vi "FPGANic-Tester.vi"() -> ()   [LabVIEW 2017]
uses:
  Source.Machine.Settings.ctl
  FPGANic.Events.ctl
  <vilib>/FPGAPlugInAG/PXIe-6592R/niLvFpga_Open_PXIe-6592R.vi
  <vilib>/rvi/interface/common/dynamic/niFpgaDynamicAddResources.vi
  <vilib>/FPGAPlugInAG/Dynamic/niLvFpga_Download_Dynamic.vi
  <vilib>/Utility/error.llb/Error Cluster From Error Code.vi
  <vilib>/rvi/errors/niLvFpgaAdjustHostInterfaceError.vi
  <vilib>/FPGAPlugInAG/Dynamic/niLvFpga_Run_Dynamic.vi
  FPGANic.Globals.vi
  <vilib>/FPGAPlugInAG/Dynamic/niLvFpga_Close_Dynamic.vi
  <vilib>/rvi/interface/nirviOpenFPGA/nirviOpenFPGA.xnode
  ProjectExportForVivado/fpga_nic/fpga_nic.lvbitx
  <vilib>/rvi/interface/nirviMethod/nirviMethod.xnode
  <vilib>/rvi/interface/nirviReadWriteControl/nirviReadWriteControl.xnode
  <vilib>/rvi/interface/nirviCloseFPGA/nirviCloseFPGA.xnode
  <vilib>/FPGAPlugInAG/Dynamic/niLvFpga_ReadFifo_Dynamic.vi
  <vilib>/rvi/errors/niLvFpgaMergeErrorWithErrorCode.vi
  <vilib>/FPGAPlugInAG/Dynamic/niLvFpga_WriteFifo_Dynamic.vi
  NiFpgaLv.dll
  <vilib>/rvi/interface/Simulation/niFpgaSimulationCallBeginRW.vi
panel:
  in  "Polling?":bool
  in  "Clear":bool
  in  "Read UART":bool
  in  "Tab Control":T1(tab)=enum."Probes/GPIO"
  in  "Ethernet II Params":T2={"Destination MAC"=[0, 2, 201, 85, 8, 68], "Source MAC"=[0, 1, 2, 3, 4, 5], "EtherType"=2048} {"Destination MAC" format="%.0x"; "Source MAC" format="%.02x"; "EtherType" format="%.0x"}
  in  "IPv4 Params":T3={"Destination IP"=[10, 0, 1, 100], "Source IP"=[10, 0, 1, 101], "Protocol"=17}
  in  "UDP Params":T4={"Source Port"=35312, "Destination Port"=35312, "Payload"="ABCD"}
  in  "MAC & IP":T5={"MAC Address"=[0, 1, 2, 3, 4, 5], "IP Address"=[10, 0, 1, 101]} {"MAC Address" format="%.0x"}
  out "Write Probe 2":u64[](array[numeric]) format="%.0x"
  out "Write Probe 1":u64[](array[numeric]) format="%.0x"
  out "Read Probe":u64[](array[numeric])=[11817445486661492224, 11817446517453291522, 11817445490022484036, 11817446517571077376, 11817445486650471966, 11817446518510649105, 11817445488139373056, 11817446517460230144, 11817445486661145833, 11817446517787656260, 11817445487417098240, 11817446519651434496, 11817445486644756480, 11817446517436909932, 11817445488513474924, 11817446519188976500, 11817445486735683427, 11817446519071309824, 11817445486669857024, 11817446517436872704, 11817445486712455169, 11817446519127149568, 11817445487441608960, 11817446517436872704, 11817445486741163008, 11817445692824123692, 11817726961621401602, 11817445490939658239, 11817446521731743746, 11817445490022484036, 11817446517571452929, 11817445486778910212, 11817446517436907522, 11817445490022484036, 11817446517604614500, 11817445486644690944, 11817446517436880915, 11817445488902144000, 11817446517436841984, 11817445486644690944, 11817446517436841984, 11817445486644690944, 11817445488835018955, 11817726961621401602, 11817445490939658239, 11817446521731743746, 11817445490022484036, 11817446517571452929, 11817445486778910212, 11817446517436907522, 11817445490022484036, 11817446517604614500, 11817445486644690944, 11817446517436895620, 11817445489682350080, 11817446517436841984, 11817445486644690944, 11817446517436841984, 11817445486644690944, 11817445488759354791, 11817726961621401602, 11817445490939658239, 11817446521731743746, 11817445490022484036, 11817446517571452929, 11817445486778910212, 11817446517436907522, 11817445490022484036, 11817446517604614500, 11817445486644690944, 11817446517436880915, 11817445488902144000, 11817446517436841984, 11817445486644690944, 11817446517436841984, 11817445486644690944, 11817445488835018955, 11817726961621401602, 11817445490939658239, 11817446521731743746, 11817445490022484036, 11817446517571452929, 11817445486778910212, 11817446517436907522, 11817445490022484036, 11817446517604614500, 11817445486644690944, 11817446517436878035, 11817445489493540864, 11817446517436841984, 11817445486644690944, 11817446517436841984, 11817445486644690944, 11817445489115705299, 11817726961621401602, 11817445490939658239, 11817446521731743746, 11817445490022484036, 11817446517571452929, 11817445486778910212, 11817446517436907522, 11817445490022484036, 11817446517604614500, 11817445486644690944, 11817446517436880915, 11817445488902144000, 11817446517436841984, 11817445486644690944, 11817446517436841984, 11817445486644690944, 11817445488835018955, 11817726961621401602, 11817445490939658239, 11817446521731743746, 11817445490022484036, 11817446517571452929, 11817445486778910212, 11817446517436907522, 11817445490022484036, 11817446517604614500, 11817445486644690944, 11817446517436878035, 11817445489493540864, 11817446517436841984, 11817445486644690944, 11817446517436841984, 11817445486644690944, 11817445489115705299, 11817726961621401602, 11817445490939658239, 11817446521731743746, 11817445490022484036, 11817446517571452929, 11817445486778910212, 11817446517436907522, 11817445490022484036, 11817446517604614500, 11817445486644690944, 11817446517436878035, 11817445489493540864, 11817446517436841984, 11817445486644690944, 11817446517436841984, 11817445486644690944, 11817445489115705299, 11817726961621401602, 11817445490939658239, 11817446521731743746, 11817445490022484036, 11817446517571452929, 11817445486778910212, 11817446517436907522, 11817445490022484036, 11817446517604614500, 11817445486644690944, 11817446517436880915, 11817445488902144000, 11817446517436841984, 11817445486644690944, 11817446517436841984, 11817445486644690944, 11817445488835018955, 11817726961621401602, 11817445486661492224, 11817446517453291522, 11817445490022484036, 11817446517571077376, 11817445486650474301, 11817446518510649105, 11817445487986346496, 11817446517460230144, 11817445486661145833, 11817446517787656260, 11817445487417098240, 11817446519651434496, 11817445486644756480, 11817446517436909932, 11817445488513474924, 11817446519188976500, 11817445486735683427, 11817446519071309824, 11817445486669857024, 11817446517436872704, 11817445486712455169, 11817446519127149568, 11817445487441608960, 11817446517436872704, 11817445486741163008, 11817445692824141017, 11817726961621401602, 11817445490939658239, 11817446521731743746, 11817445490022484036, 11817446517571452929, 11817445486778910212, 11817446517436907522, 11817445490022484036, 11817446517604614500, 11817445486644690944, 11817446517436878035, 11817445489493540864, 11817446517436841984, 11817445486644690944, 11817446517436841984, 11817445486644690944, 11817445489115705299, 11817726961621401602, 11817445490939658239, 11817446521731743746, 11817445490022484036, 11817446517571452929, 11817445486778910212, 11817446517436907522, 11817445490022484036, 11817446517604614500, 11817445486644690944, 11817446517436859339, 11817445486682636288, 11817446517436841984, 11817445486644690944, 11817446517436841984, 11817445486644690944, 11817445488555902218, 11817726961621401602, 11817445490939658239, 11817446521731743746, 11817445490022484036, 11817446517571452929, 11817445486778910212, 11817446517436907522, 11817445490022484036, 11817446517604614500, 11817445486644690944, 11817446517436859339, 11817445486682636288, 11817446517436841984, 11817445486644690944, 11817446517436841984, 11817445486644690944, 11817445488555902218, 11817726961621401602, 11817445490939658239, 11817446521731743746, 11817445490022484036, 11817446517571452929, 11817445486778910212, 11817446517436907522, 11817445490022484036, 11817446517604614500, 11817445486644690944, 11817446517436878035, 11817445489493540864, 11817446517436841984, 11817445486644690944, 11817446517436841984, 11817445486644690944, 11817445489115705299, 11817726961621401602, 11817445490939658239, 11817446521731743746, 11817445490022484036, 11817446517571452929, 11817445486778910212, 11817446517436907522, 11817445490022484036, 11817446517604614500, 11817445486644690944, 11817446517436878035, 11817445489493540864, 11817446517436841984, 11817445486644690944, 11817446517436841984, 11817445486644690944, 11817445489115705299, 11817726961621401602, 11817445490939658239, 11817446521731743746, 11817445490022484036, 11817446517571452929, 11817445486778910212, 11817446517436907522, 11817445490022484036, 11817446517604614500, 11817445486644690944, 11817446517436859339, 11817445486682636288, 11817446517436841984, 11817445486644690944, 11817446517436841984, 11817445486644690944, 11817445488555902218, 11817726961621401602, 11817445490939658239, 11817446521731743746, 11817445490022484036, 11817446517571452929, 11817445486778910212, 11817446517436907522, 11817445490022484036, 11817446517604614500, 11817445486644690944, 11817446517436859339, 11817445486682636288, 11817446517436841984, 11817445486644690944, 11817446517436841984, 11817445486644690944, 11817445488555902218, 11817726961621401602, 11817445490939658239, 11817446521731743746, 11817445490022484036, 11817446517571452929, 11817445486778910212, 11817446517436907522, 11817445490022484036, 11817446517604614500, 11817445486644690944, 11817446517436844075, 11817445488075145216, 11817446517436841984, 11817445486644690944, 11817446517436841984, 11817445486644690944, 11817445490337402917, 11817726961621401602, 11817445490939658239, 11817446521731743746, 11817445490022484036, 11817446517571452929, 11817445486778910212, 11817446517436907522, 11817445490022484036, 11817446517604614500, 11817445486644690944, 11817446517436859339, 11817445486682636288, 11817446517436841984, 11817445486644690944, 11817446517436841984, 11817445486644690944, 11817445488555902218, 11817726961621401602, 11817445490939658239, 11817446521731743746, 11817445490022484036, 11817446517571452929, 11817445486778910212, 11817446517436907522, 11817445490022484036, 11817446517604614500, 11817445486644690944, 11817446517436844075, 11817445488075145216, 11817446517436841984, 11817445486644690944, 11817446517436841984, 11817445486644690944, 11817445490337402917, 11817726961621401602, 11817445490939658239, 11817446521731743746, 11817445490022484036, 11817446517571452929, 11817445486778910212, 11817446517436907522, 11817445490022484036, 11817446517604614500, 11817445486644690944, 11817446517436859339, 11817445486682636288, 11817446517436841984, 11817445486644690944, 11817446517436841984, 11817445486644690944, 11817445488555902218, 11817726961621401602, 11817445490939658239, 11817446521731743746, 11817445490022484036, 11817446517571452929, 11817445486778910212, 11817446517436907522, 11817445490022484036, 11817446517604614500, 11817445486644690944, 11817446517436844075, 11817445488075145216, 11817446517436841984, 11817445486644690944, 11817446517436841984, 11817445486644690944, 11817445490337402917, 11817726961621401602, 11817445490939658239, 11817446521731743746, 11817445490022484036, 11817446517571452929, 11817445486778910212, 11817446517436907522, 11817445490022484036, 11817446517604614500, 11817445486644690944, 11817446517436844075, 11817445488075145216, 11817446517436841984, 11817445486644690944, 11817446517436841984, 11817445486644690944, 11817445490337402917, 11817726961621401602, 11817445490939658239, 11817446521731743746, 11817445490022484036, 11817446517571452929, 11817445486778910212, 11817446517436907522, 11817445490022484036, 11817446517604614500, 11817445486644690944, 11817446517436880915, 11817445488905814016, 11817446517436841984, 11817445486644690944, 11817446517436841984, 11817445486644690944, 11817445487441373583, 11817726961621401602, 11817445490939658239, 11817446521731743746, 11817445490022484036, 11817446517571452929, 11817445486778910212, 11817446517436907522, 11817445490022484036, 11817446517604614500, 11817445486644690944, 11817446517436844075, 11817445488075145216, 11817446517436841984, 11817445486644690944, 11817446517436841984, 11817445486644690944, 11817445490337402917, 11817726961621401602, 11817445490939658239, 11817446521731743746, 11817445490022484036, 11817446517571452929, 11817445486778910212, 11817446517436907522, 11817445490022484036, 11817446517604614500, 11817445486644690944, 11817446517436880915, 11817445488905814016, 11817446517436841984, 11817445486644690944, 11817446517436841984, 11817445486644690944, 11817445487441373583, 11817726961621401602, 11817445486661492224, 11817446517453291522, 11817445490022484036, 11817446517571077376, 11817445486650478677, 11817446518510649105, 11817445487699560960, 11817446517460230144, 11817445486661145833, 11817446517787656260, 11817445487417098240, 11817446519651434496, 11817445486644756480, 11817446517436909932, 11817445488513474924, 11817446519188976500, 11817445486735683427, 11817446519071309824, 11817445486669857024, 11817446517436872704, 11817445486712455169, 11817446519127149568, 11817445487441608960, 11817446517436872704, 11817445486741163008, 11817445692824141166, 11817726961621401602, 11817445490939658239, 11817446521731743746, 11817445490022484036, 11817446517571452929, 11817445486778910212, 11817446517436907522, 11817445490022484036, 11817446517604614500, 11817445486644690944, 11817446517436844075, 11817445488075145216, 11817446517436841984, 11817445486644690944, 11817446517436841984, 11817445486644690944, 11817445490337402917, 11817726961621401602, 11817445490939658239, 11817446521731743746, 11817445490022484036, 11817446517571452929, 11817445486778910212, 11817446517436907522, 11817445490022484036, 11817446517604614500, 11817445486644690944, 11817446517436880915, 11817445488905814016, 11817446517436841984, 11817445486644690944, 11817446517436841984, 11817445486644690944, 11817445487441373583, 11817726961621401602, 11817445490939658239, 11817446521731743746, 11817445490022484036, 11817446517571452929, 11817445486778910212, 11817446517436907522, 11817445490022484036, 11817446517604614500, 11817445486644690944, 11817446517436880915, 11817445488905814016, 11817446517436841984, 11817445486644690944, 11817446517436841984, 11817445486644690944, 11817445487441373583, 11817726961621401602, 11817445490939658239, 11817446521731743746, 11817445490022484036, 11817446517571452929, 11817445486778910212, 11817446517436907522, 11817445490022484036, 11817446517604614500, 11817445486644690944, 11817446517436859355, 11817445489065066496, 11817446517436841984, 11817445486644690944, 11817446517436841984, 11817445486644690944, 11817445488052856394, 11817726961621401602, 11817445490939658239, 11817446521731743746, 11817445490022484036, 11817446517571452929, 11817445486778910212, 11817446517436907522, 11817445490022484036, 11817446517604614500, 11817445486644690944, 11817446517436880915, 11817445488905814016, 11817446517436841984, 11817445486644690944, 11817446517436841984, 11817445486644690944, 11817445487441373583, 11817726961621401602, 11817445490939658239, 11817446521731743746, 11817445490022484036, 11817446517571452929, 11817445486778910212, 11817446517436907522, 11817445490022484036, 11817446517604614500, 11817445486644690944, 11817446517436859355, 11817445489065066496, 11817446517436841984, 11817445486644690944, 11817446517436841984, 11817445486644690944, 11817445488052856394, 11817726961621401602, 11817445490939658239, 11817446521731743746, 11817445490022484036, 11817446517571452929, 11817445486778910212, 11817446517436907522, 11817445490022484036, 11817446517604614500, 11817445486644690944, 11817446517436859355, 11817445489065066496, 11817446517436841984, 11817445486644690944, 11817446517436841984, 11817445486644690944, 11817445488052856394, 11817726961621401602, 11817445490939658239, 11817446521731743746, 11817445490022484036, 11817446517571452929, 11817445486778910212, 11817446517436907522, 11817445490022484036, 11817446517604614500, 11817445486644690944, 11817446517436880915, 11817445488905814016, 11817446517436841984, 11817445486644690944, 11817446517436841984, 11817445486644690944, 11817445487441373583, 11817726961621401602, 11817445490939658239, 11817446521731743746, 11817445490022484036, 11817446517571452929, 11817445486778910212, 11817446517436907522, 11817445490022484036, 11817446517604614500, 11817445486644690944, 11817446517436859355, 11817445489065066496, 11817446517436841984, 11817445486644690944, 11817446517436841984, 11817445486644690944, 11817445488052856394, 11817726961621401602, 11817445490939658239, 11817446521731743746, 11817445490022484036, 11817446517571452929, 11817445486778910212, 11817446517436907522, 11817445490022484036, 11817446517604614500, 11817445486644690944, 11817446517436878035, 11817445489492885504, 11817446517436841984, 11817445486644690944, 11817446517436841984, 11817445486644690944, 11817445490525715118, 11817726961621401602, 11817445490939658239, 11817446521731743746, 11817445490022484036, 11817446517571452929, 11817445486778910212, 11817446517436907522, 11817445490022484036, 11817446517604614500, 11817445486644690944, 11817446517436878035, 11817445489492885504, 11817446517436841984, 11817445486644690944, 11817446517436841984, 11817445486644690944, 11817445490525715118, 11817726961621401602, 11817445490939658239, 11817446521731743746, 11817445490022484036, 11817446517571452929, 11817445486778910212, 11817446517436907522, 11817445490022484036, 11817446517604614500, 11817445486644690944, 11817446517436859355, 11817445489065066496, 11817446517436841984, 11817445486644690944, 11817446517436841984, 11817445486644690944, 11817445488052856394, 11817726961621401602, 11817445490939658239, 11817446521731743746, 11817445490022484036, 11817446517571452929, 11817445486778910212, 11817446517436907522, 11817445490022484036, 11817446517604614500, 11817445486644690944, 11817446517436859355, 11817445489065066496, 11817446517436841984, 11817445486644690944, 11817446517436841984, 11817445486644690944, 11817445488052856394, 11817726961621401602, 11817445490939658239, 11817446521731743746, 11817445490022484036, 11817446517571452929, 11817445486778910212, 11817446517436907522, 11817445490022484036, 11817446517604614500, 11817445486644690944, 11817446517436878035, 11817445489492885504, 11817446517436841984, 11817445486644690944, 11817446517436841984, 11817445486644690944, 11817445490525715118, 11817726961621401602, 11817445490939658239, 11817446521731743746, 11817445490022484036, 11817446517571452929, 11817445486778910212, 11817446517436907522, 11817445490022484036, 11817446517604614500, 11817445486644690944, 11817446517436878035, 11817445489492885504, 11817446517436841984, 11817445486644690944, 11817446517436841984, 11817445486644690944, 11817445490525715118, 11817726961621401602, 11817445490939658239, 11817446521731743746, 11817445490022484036, 11817446517571452929, 11817445486778910212, 11817446517436907522, 11817445490022484036, 11817446517604614500, 11817445486644690944, 11817446517436858915, 11817445487695495168, 11817446517436841984, 11817445486644690944, 11817446517436841984, 11817445486644690944, 11817445489806603878, 11817726961621401602, 11817445490939658239, 11817446521731743746, 11817445490022484036, 11817446517571452929, 11817445486778910212, 11817446517436907522, 11817445490022484036, 11817446517604614500, 11817445486644690944, 11817446517436878035, 11817445489492885504, 11817446517436841984, 11817445486644690944, 11817446517436841984, 11817445486644690944, 11817445490525715118, 11817726961621401602, 11817445490939658239, 11817446521731743746, 11817445490022484036, 11817446517571452929, 11817445486778910212, 11817446517436907522, 11817445490022484036, 11817446517604614500, 11817445486644690944, 11817446517436858915, 11817445487695495168, 11817446517436841984, 11817445486644690944, 11817446517436841984, 11817445486644690944, 11817445489806603878, 11817726961621401602, 11817445486661492224, 11817446517453291522, 11817445490022484036, 11817446517571077376, 11817445486649761975, 11817446518510649105, 11817445487425423872, 11817446517460230144, 11817445486661145833, 11817446517787656249, 11817445488492281856, 11817446517436841985, 11817445486644690945, 11817446517436844396, 11817445488513474924, 11817446519188976500, 11817445486735683427, 11817446519071309824, 11817445490922881472, 11817446517638168832, 11817445486661468160, 11817446519450108938, 11817445486644782091, 11817445453811713277, 11817726961621401602, 11817445486661492224, 11817446517453291522, 11817445490022484036, 11817446517571077376, 11817445486649762087, 11817446518510649105, 11817445487418083840, 11817446517460230144, 11817445486661145833, 11817446517787656249, 11817445488492281856, 11817446517436841985, 11817445486644690945, 11817446517436844396, 11817445488513474924, 11817446519188976500, 11817445486735683427, 11817446519071309824, 11817445490922881472, 11817446517638168832, 11817445486661468160, 11817446519450108938, 11817445486644782266, 11817445452738132989, 11817726961621401602, 11817445490939658239, 11817446521731743746, 11817445490022484036, 11817446517571452929, 11817445486778910212, 11817446517436907522, 11817445490022484036, 11817446517604614500, 11817445486644690944, 11817446517436878035, 11817445489492885504, 11817446517436841984, 11817445486644690944, 11817446517436841984, 11817445486644690944, 11817445490525715118, 11817726961621401602, 11817445490939658239, 11817446521731743746, 11817445490022484036, 11817446517571452929, 11817445486778910212, 11817446517436907522, 11817445490022484036, 11817446517604614500, 11817445486644690944, 11817446517436858915, 11817445487695495168, 11817446517436841984, 11817445486644690944, 11817446517436841984, 11817445486644690944, 11817445489806603878, 11817726961621401602, 11817445486661492224, 11817446517453291522, 11817445490022484036, 11817446517571077376, 11817445486649762234, 11817446518510649105, 11817445487408450048, 11817446517460230144, 11817445486661145833, 11817446517787656249, 11817445488492281856, 11817446517436841985, 11817445486644690945, 11817446517436844396, 11817445488513474924, 11817446519188976500, 11817445486735683427, 11817446519071309824, 11817445490922881472, 11817446517638168832, 11817445486661468160, 11817446519450108938, 11817445486644782315, 11817445454750429437, 11817726961621401602, 11817445486661492224, 11817446517453291522, 11817445490022484036, 11817446517571077376, 11817445486652908126, 11817446518510649105, 11817445487394556416, 11817446517460230144, 11817445486661145833, 11817446517787656297, 11817445488489922560, 11817446519651434496, 11817445486644822016, 11817446517436909932, 11817445488513474924, 11817446519188976500, 11817445486735683427, 11817446519071309824, 11817445486669857024, 11817446517436872704, 11817445486712455169, 11817446519114772784, 11817445487450075393, 11817446518242292016, 11817445486769040941, 11817446519070811250, 11817445486718186096, 11817446519064231948, 11817445488792240128, 11817446517444706306, 11817445489866752012, 11817446517439954945, 11817445486644691064, 11817446517437218828, 11817445486644773000, 11817445453377722877, 11817726961621401602, 11817445486661492224, 11817446517453291522, 11817445490022484036, 11817446517571077376, 11817445486651073205, 11817446518510649105, 11817445487390689792, 11817446517460230144, 11817445486661145833, 11817446517787656269, 11817445487799631872, 11817446517436841985, 11817445486644690945, 11817446517436842801, 11817445487453143345, 11817446517456765489, 11817445487450483054, 11817446518198199396, 11817445488557580658, 11817446519322247168, 11817445490922881472, 11817446517638171648, 11817445486661468160, 11817446519450112008, 11817445488463539829, 11817446519453069873, 11817445486735683427, 11817445969315496190, 11817726961621401602, 11817445486661492224, 11817446517453291522, 11817445490022484036, 11817446517571077376, 11817445486651073370, 11817446518510649105, 11817445487379876352, 11817446517460230144, 11817445486661145833, 11817446517787656269, 11817445487799631872, 11817446517436841985, 11817445486644690945, 11817446517436842801, 11817445487453143345, 11817446517456765489, 11817445487450483054, 11817446518198199396, 11817445488557580658, 11817446519322247168, 11817445490922881472, 11817446517638171648, 11817445486661468160, 11817446519450112008, 11817445488463539829, 11817446519453069873, 11817445486735683427, 11817445969315496167, 11817726961621401602, 11817445486661492224, 11817446517453291522, 11817445490022484036, 11817446517571077376, 11817445486651073405, 11817446518510649105, 11817445487377582592, 11817446517460230144, 11817445486661145833, 11817446517787656269, 11817445487799631872, 11817446517436841985, 11817445486644690945, 11817446517436842801, 11817445487453143345, 11817446517456765489, 11817445487450483054, 11817446518198199396, 11817445488557580658, 11817446519322247168, 11817445490922881472, 11817446517638171648, 11817445486661468160, 11817446519450112008, 11817445488463539829, 11817446519453069873, 11817445486735683427, 11817445969315495936, 11817726961621401602, 11817445486661492224, 11817446517453291522, 11817445490022484036, 11817446517571077376, 11817445486650680210, 11817446518510649105, 11817445487376599552, 11817446517460230144, 11817445486661145833, 11817446517787656263, 11817445490086379520, 11817446519651434496, 11817445486644756480, 11817446517436842801, 11817445487453143345, 11817446517456765489, 11817445487450483054, 11817446518198199396, 11817445488557580658, 11817446519322247168, 11817445486854406400, 11817446517436872704, 11817445486913678441, 11817446519290034221, 11817445487486764396, 11817446519305625964, 11817445486650109318, 11817445428830209799, 11817726961621401602, 11817445486661492224, 11817446517453291522, 11817445490022484036, 11817446517571077376, 11817445486650483777, 11817446518510649105, 11817445487365327360, 11817446517460230144, 11817445486661145833, 11817446517787656260, 11817445487417098240, 11817446519651434496, 11817445486644756480, 11817446517436909932, 11817445488513474924, 11817446519188976500, 11817445486735683427, 11817446519071309824, 11817445486669857024, 11817446517436872704, 11817445486712455169, 11817446519127149568, 11817445487441608960, 11817446517436872704, 11817445486741163008, 11817445692824112747, 11817726961621401602, 11817445486661492224, 11817446517453291522, 11817445490022484036, 11817446517571077376, 11817445486650674912, 11817446518510649105, 11817445487723809280, 11817446517460230144, 11817445486661145833, 11817446517787656263, 11817445490086379520, 11817446519651434496, 11817445486644756480, 11817446517436842801, 11817445487453143345, 11817446517456765489, 11817445487450483054, 11817446518198199396, 11817445488557580658, 11817446519322247168, 11817445486854406400, 11817446517436872704, 11817445486913678441, 11817446519290034221, 11817445487486764396, 11817446519305625964, 11817445486652761861, 11817445427538364167, 11817726961621401602, 11817445490939658239, 11817446521731743746, 11817445490022484036, 11817446517571452929, 11817445486778910212, 11817446517436907522, 11817445490022484036, 11817446517604614500, 11817445486644690944, 11817446517436878035, 11817445489492885504, 11817446517436841984, 11817445486644690944, 11817446517436841984, 11817445486644690944, 11817445490525715118, 11817726961621401602, 11817445490939658239, 11817446521731743746, 11817445490022484036, 11817446517571452929, 11817445486778910212, 11817446517436907522, 11817445490022484036, 11817446517604614500, 11817445486644690944, 11817446517436844075, 11817445488075145216, 11817446517436841984, 11817445486644690944, 11817446517436841984, 11817445486644690944, 11817445490337402917, 11817726961621401602, 11817445486661492224, 11817446517453291522, 11817445490022484036, 11817446517571077376, 11817445486650478551, 11817446518510649105, 11817445487707818496, 11817446517460230144, 11817445486661145833, 11817446517787656260, 11817445487417098240, 11817446519651434496, 11817445486644756480, 11817446517436909932, 11817445488513474924, 11817446519188976500, 11817445486735683427, 11817446519071309824, 11817445486669857024, 11817446517436872704, 11817445486712455169, 11817446519127149568, 11817445487441608960, 11817446517436872704, 11817445486741163008, 11817445692824104959, 11817726961621401602, 11817445490939658239, 11817446521731743746, 11817445490022484036, 11817446517571452929, 11817445486778910212, 11817446517436907522, 11817445490022484036, 11817446517604614500, 11817445486644690944, 11817446517436844075, 11817445488075145216, 11817446517436841984, 11817445486644690944, 11817446517436841984, 11817445486644690944, 11817445490337402917, 11817726961621401602, 11817445490939658239, 11817446521731743746, 11817445490022484036, 11817446517571452929, 11817445486778910212, 11817446517436907522, 11817445490022484036, 11817446517604614500, 11817445486644690944, 11817446517436880915, 11817445488905814016, 11817446517436841984, 11817445486644690944, 11817446517436841984, 11817445486644690944, 11817445487441373583, 11817726961621401602, 11817445486661492224, 11817446517453291522, 11817445490022484036, 11817446517571077376, 11817445486650675876, 11817446518510649105, 11817445487660632576, 11817446517460230144, 11817445486661145833, 11817446517787656263, 11817445490086379520, 11817446519651434496, 11817445486644756480, 11817446517436842801, 11817445487453143345, 11817446517456765489, 11817445487450483054, 11817446518198199396, 11817445488557580658, 11817446519322247168, 11817445486854406400, 11817446517436872704, 11817445486913678441, 11817446519290034221, 11817445487486764396, 11817446519305625964, 11817445486655633830, 11817445428595328775, 11817726961621401602, 11817445490939658239, 11817446521731743746, 11817445490022484036, 11817446517571452929, 11817445486778910212, 11817446517436907522, 11817445490022484036, 11817446517604614500, 11817445486644690944, 11817446517436880915, 11817445488905814016, 11817446517436841984, 11817445486644690944, 11817446517436841984, 11817445486644690944, 11817445487441373583, 11817726961621401602, 11817445490939658239, 11817446521731743746, 11817445490022484036, 11817446517571452929, 11817445486778910212, 11817446517436907522, 11817445490022484036, 11817446517604614500, 11817445486644690944, 11817446517436844075, 11817445488075145216, 11817446517436841984, 11817445486644690944, 11817446517436841984, 11817445486644690944, 11817445490337402917, 11817726961621401602, 11817445490939658239, 11817446521731743746, 11817445490022484036, 11817446517571452929, 11817445486778910212, 11817446517436907522, 11817445490022484036, 11817446517604614500, 11817445486644690944, 11817446517436844075, 11817445488075145216, 11817446517436841984, 11817445486644690944, 11817446517436841984, 11817445486644690944, 11817445490337402917, 11817726961621401602, 11817445490939658239, 11817446521731743746, 11817445490022484036, 11817446517571452929, 11817445486778910212, 11817446517436907522, 11817445490022484036, 11817446517604614500, 11817445486644690944, 11817446517436880915, 11817445488905814016, 11817446517436841984, 11817445486644690944, 11817446517436841984, 11817445486644690944, 11817445487441373583, 11817726961621401602, 11817445490939658239, 11817446521731743746, 11817445490022484036, 11817446517571452929, 11817445486778910212, 11817446517436907522, 11817445490022484036, 11817446517604614500, 11817445486644690944, 11817446517436880915, 11817445488905814016, 11817446517436841984, 11817445486644690944, 11817446517436841984, 11817445486644690944, 11817445487441373583, 11817726961621401602, 11817445490939658239, 11817446521731743746, 11817445490022484036, 11817446517571452929, 11817445486778910212, 11817446517436907522, 11817445490022484036, 11817446517604614500, 11817445486644690944, 11817446517436878035, 11817445489493540864, 11817446517436841984, 11817445486644690944, 11817446517436841984, 11817445486644690944, 11817445489115705299, 11817726961621401602, 11817445486661492224, 11817446517453291522, 11817445490022484036, 11817446517571077376, 11817445486650481225, 11817446518510649105, 11817445487532575232, 11817446517460230144, 11817445486661145833, 11817446517787656260, 11817445487417098240, 11817446519651434496, 11817445486644756480, 11817446517436909932, 11817445488513474924, 11817446519188976500, 11817445486735683427, 11817446519071309824, 11817445486669857024, 11817446517436872704, 11817445486712455169, 11817446519127149568, 11817445487441608960, 11817446517436872704, 11817445486741163008, 11817445692824103053, 11817726961621401602, 11817445490939658239, 11817446521731743746, 11817445490022484036, 11817446517571452929, 11817445486778910212, 11817446517436907522, 11817445490022484036, 11817446517604614500, 11817445486644690944, 11817446517436880915, 11817445488905814016, 11817446517436841984, 11817445486644690944, 11817446517436841984, 11817445486644690944, 11817445487441373583, 11817726961621401602, 11817445490939658239, 11817446521731743746, 11817445490022484036, 11817446517571452929, 11817445486778910212, 11817446517436907522, 11817445490022484036, 11817446517604614500, 11817445486644690944, 11817446517436878035, 11817445489493540864, 11817446517436841984, 11817445486644690944, 11817446517436841984, 11817445486644690944, 11817445489115705299, 11817726961621401602, 11817445490939658239, 11817446521731743746, 11817445490022484036, 11817446517571452929, 11817445486778910212, 11817446517436907522, 11817445490022484036, 11817446517604614500, 11817445486644690944, 11817446517436878035, 11817445489493540864, 11817446517436841984, 11817445486644690944, 11817446517436841984, 11817445486644690944, 11817445489115705299, 11817726961621401602, 11817445490939658239, 11817446521731743746, 11817445490022484036, 11817446517571452929, 11817445486778910212, 11817446517436907522, 11817445490022484036, 11817446517604614500, 11817445486644690944, 11817446517436880915, 11817445488905814016, 11817446517436841984, 11817445486644690944, 11817446517436841984, 11817445486644690944, 11817445487441373583, 11817726961621401602, 11817445490939658239, 11817446521731743746, 11817445490022484036, 11817446517571452929, 11817445486778910212, 11817446517436907522, 11817445490022484036, 11817446517604614500, 11817445486644690944, 11817446517436878035, 11817445489493540864, 11817446517436841984, 11817445486644690944, 11817446517436841984, 11817445486644690944, 11817445489115705299, 11817726961621401602, 11817445490939658239, 11817446521731743746, 11817445490022484036, 11817446517571452929, 11817445486778910212, 11817446517436907522, 11817445490022484036, 11817446517604614500, 11817445486644690944, 11817446517436889485, 11817445489429577728, 11817446517436841984, 11817445486644690944, 11817446517436841984, 11817445486644690944, 11817445488947655731, 11817726961621401602, 11817445490939658239, 11817446521731743746, 11817445490022484036, 11817446517571452929, 11817445486778910212, 11817446517436907522, 11817445490022484036, 11817446517604614500, 11817445486644690944, 11817446517436889485, 11817445489429577728, 11817446517436841984, 11817445486644690944, 11817446517436841984, 11817445486644690944, 11817445488947655731, 11817726961621401602, 11817445490939658239, 11817446521731743746, 11817445490022484036, 11817446517571452929, 11817445486778910212, 11817446517436907522, 11817445490022484036, 11817446517604614500, 11817445486644690944, 11817446517436878035, 11817445489493540864, 11817446517436841984, 11817445486644690944, 11817446517436841984, 11817445486644690944, 11817445489115705299, 11817726961621401602, 11817445490939658239, 11817446521731743746, 11817445490022484036, 11817446517571452929, 11817445486778910212, 11817446517436907522, 11817445490022484036, 11817446517604614500, 11817445486644690944, 11817446517436878035, 11817445489493540864, 11817446517436841984, 11817445486644690944, 11817446517436841984, 11817445486644690944, 11817445489115705299, 11817726961621401602, 11817445490939658239, 11817446521731743746, 11817445490022484036, 11817446517571452929, 11817445486778910212, 11817446517436907522, 11817445490022484036, 11817446517604614500, 11817445486644690944, 11817446517436889485, 11817445489429577728, 11817446517436841984, 11817445486644690944, 11817446517436841984, 11817445486644690944, 11817445488947655731, 11817726961621401602, 11817445490939658239, 11817446521731743746, 11817445490022484036, 11817446517571452929, 11817445486778910212, 11817446517436907522, 11817445490022484036, 11817446517604614500, 11817445486644690944, 11817446517436889485, 11817445489429577728, 11817446517436841984, 11817445486644690944, 11817446517436841984, 11817445486644690944, 11817445488947655731, 11817726961621401602, 11817445490939658239, 11817446521731743746, 11817445490022484036, 11817446517571452929, 11817445486778910212, 11817446517436907522, 11817445490022484036, 11817446517604614500, 11817445486644690944, 11817446517436895620, 11817445489682350080, 11817446517436841984, 11817445486644690944, 11817446517436841984, 11817445486644690944, 11817445488759354791, 11817726961621401602, 11817445490939658239, 11817446521731743746, 11817445490022484036, 11817446517571452929, 11817445486778910212, 11817446517436907522, 11817445490022484036, 11817446517604614500, 11817445486644690944, 11817446517436889485, 11817445489429577728, 11817446517436841984, 11817445486644690944, 11817446517436841984, 11817445486644690944, 11817445488947655731, 11817726961621401602, 11817445490939658239, 11817446521731743746, 11817445490022484036, 11817446517571452929, 11817445486778910212, 11817446517436907522, 11817445490022484036, 11817446517604614500, 11817445486644690944, 11817446517436895620, 11817445489682350080, 11817446517436841984, 11817445486644690944, 11817446517436841984, 11817445486644690944, 11817445488759354791, 11817726961621401602, 11817445490939658239, 11817446521731743746, 11817445490022484036, 11817446517571452929, 11817445486778910212, 11817446517436907522, 11817445490022484036, 11817446517604614500, 11817445486644690944, 11817446517436895620, 11817445489682350080, 11817446517436841984, 11817445486644690944, 11817446517436841984, 11817445486644690944, 11817445488759354791, 11817726961621401602, 11817445490939658239, 11817446521731743746, 11817445490022484036, 11817446517571452929, 11817445486778910212, 11817446517436907522, 11817445490022484036, 11817446517604614500, 11817445486644690944, 11817446517436889485, 11817445489429577728, 11817446517436841984, 11817445486644690944, 11817446517436841984, 11817445486644690944, 11817445488947655731, 11817726961621401602, 11817445486661492224, 11817446517453291522, 11817445490022484036, 11817446517571077376, 11817445486650485803, 11817446518510649105, 11817445487232551424, 11817446517460230144, 11817445486661145833, 11817446517787656260, 11817445487417098240, 11817446519651434496, 11817445486644756480, 11817446517436909932, 11817445488513474924, 11817446519188976500, 11817445486735683427, 11817446519071309824, 11817445486669857024, 11817446517436872704, 11817445486712455169, 11817446519127149568, 11817445487441608960, 11817446517436872704, 11817445486741163008, 11817445692824156020, 11817726961621401602, 11817445490939658239, 11817446521731743746, 11817445490022484036, 11817446517571452929, 11817445486778910212, 11817446517436907522, 11817445490022484036, 11817446517604614500, 11817445486644690944, 11817446517436895620, 11817445489682350080, 11817446517436841984, 11817445486644690944, 11817446517436841984, 11817445486644690944, 11817445488759354791, 11817726961621401602, 11817445490939658239, 11817446521731743746, 11817445490022484036, 11817446517571452929, 11817445486778910212, 11817446517436907522, 11817445490022484036, 11817446517604614500, 11817445486644690944, 11817446517436880915, 11817445488902144000, 11817446517436841984, 11817445486644690944, 11817446517436841984, 11817445486644690944, 11817445488835018955, 11817726961621401602, 11817445490939658239, 11817446521731743746, 11817445490022484036, 11817446517571452929, 11817445486778910212, 11817446517436907522, 11817445490022484036, 11817446517604614500, 11817445486644690944, 11817446517436880915, 11817445488902144000, 11817446517436841984, 11817445486644690944, 11817446517436841984, 11817445486644690944, 11817445488835018955, 11817726961621401602, 11817445490939658239, 11817446521731743746, 11817445490022484036, 11817446517571452929, 11817445486778910212, 11817446517436907522, 11817445490022484036, 11817446517604614500, 11817445486644690944, 11817446517436895620, 11817445489682350080, 11817446517436841984, 11817445486644690944, 11817446517436841984, 11817445486644690944, 11817445488759354791, 11817726961621401602, 11817445490939658239, 11817446521731743746, 11817445490022484036, 11817446517571452929, 11817445486778910212, 11817446517436907522, 11817445490022484036, 11817446517604614500, 11817445486644690944, 11817446517436895620, 11817445489682350080, 11817446517436841984, 11817445486644690944, 11817446517436841984, 11817445486644690944, 11817445488759354791, 11817726961621401602, 11817445490939658239, 11817446521731743746, 11817445490022484036, 11817446517571452929, 11817445486778910212, 11817446517436907522, 11817445490022484036, 11817446517604614500, 11817445486644690944, 11817446517436880915, 11817445488902144000, 11817446517436841984, 11817445486644690944, 11817446517436841984, 11817445486644690944, 11817445488835018955, 11817726961621401602, 11817445490939658239, 11817446521731743746, 11817445490022484036, 11817446517571452929, 11817445486778910212, 11817446517436907522, 11817445490022484036, 11817446517604614500, 11817445486644690944, 11817446517436880915, 11817445488902144000, 11817446517436841984, 11817445486644690944, 11817446517436841984, 11817445486644690944, 11817445488835018955, 11817726961621401602, 11817445490939658239, 11817446521731743746, 11817445490022484036, 11817446517571452929, 11817445486778910212, 11817446517436907522, 11817445490022484036, 11817446517604614500, 11817445486644690944, 11817446517436859355, 11817445489065066496, 11817446517436841984, 11817445486644690944, 11817446517436841984, 11817445486644690944, 11817445488052856394, 11817726961621401602, 11817445490939658239, 11817446521731743746, 11817445490022484036, 11817446517571452929, 11817445486778910212, 11817446517436907522, 11817445490022484036, 11817446517604614500, 11817445486644690944, 11817446517436859355, 11817445489065066496, 11817446517436841984, 11817445486644690944, 11817446517436841984, 11817445486644690944, 11817445488052856394, 11817726961621401602, 11817445490939658239, 11817446521731743746, 11817445490022484036, 11817446517571452929, 11817445486778910212, 11817446517436907522, 11817445490022484036, 11817446517604614500, 11817445486644690944, 11817446517436880915, 11817445488902144000, 11817446517436841984, 11817445486644690944, 11817446517436841984, 11817445486644690944, 11817445488835018955, 11817726961621401602, 11817445490939658239, 11817446521731743746, 11817445490022484036, 11817446517571452929, 11817445486778910212, 11817446517436907522, 11817445490022484036, 11817446517604614500, 11817445486644690944, 11817446517436880915, 11817445488902144000, 11817446517436841984, 11817445486644690944, 11817446517436841984, 11817445486644690944, 11817445488835018955, 11817726961621401602, 11817445490939658239, 11817446521731743746, 11817445490022484036, 11817446517571452929, 11817445486778910212, 11817446517436907522, 11817445490022484036, 11817446517604614500, 11817445486644690944, 11817446517436859355, 11817445489065066496, 11817446517436841984, 11817445486644690944, 11817446517436841984, 11817445486644690944, 11817445488052856394, 11817726961621401602, 11817445490939658239, 11817446521731743746, 11817445490022484036, 11817446517571452929, 11817445486778910212, 11817446517436907522, 11817445490022484036, 11817446517604614500, 11817445486644690944, 11817446517436859355, 11817445489065066496, 11817446517436841984, 11817445486644690944, 11817446517436841984, 11817445486644690944, 11817445488052856394, 11817726961621401602, 11817445490939658239, 11817446521731743746, 11817445490022484036, 11817446517571452929, 11817445486778910212, 11817446517436907522, 11817445490022484036, 11817446517604614500, 11817445486644690944, 11817446517436859355, 11817445489065066496, 11817446517436841984, 11817445486644690944, 11817446517436841984, 11817445486644690944, 11817445488052856394, 11817726961621401602, 11817445490939658239, 11817446521731743746, 11817445490022484036, 11817446517571452929, 11817445486778910212, 11817446517436907522, 11817445490022484036, 11817446517604614500, 11817445486644690944, 11817446517436859355, 11817445489065066496, 11817446517436841984, 11817445486644690944, 11817446517436841984, 11817445486644690944, 11817445488052856394, 11817726961621401602, 11817445486661492224, 11817446517453291522, 11817445490022484036, 11817446517571077376, 11817445486650497716, 11817446518510649105, 11817445490746722816, 11817446517460230144, 11817445486661145833, 11817446517787656260, 11817445487417098240, 11817446519651434496, 11817445486644756480, 11817446517436909932, 11817445488513474924, 11817446519188976500, 11817445486735683427, 11817446519071309824, 11817445486669857024, 11817446517436872704, 11817445486712455169, 11817446519127149568, 11817445487441608960, 11817446517436872704, 11817445486741163008, 11817445692824105340, 11817726961621401602, 11817445490939658239, 11817446521731743746, 11817445490022484036, 11817446517571452929, 11817445486778910212, 11817446517436907522, 11817445490022484036, 11817446517604614500, 11817445486644690944, 11817446517436844544, 11817445486668087296, 11817446517436841984, 11817445486644690944, 11817446517436841984, 11817445486644690944, 11817445488739790818, 11817726961621401602, 11817445490939658239, 11817446521731743746, 11817445490022484036, 11817446517571452929, 11817445486778910212, 11817446517436907522, 11817445490022484036, 11817446517604614500, 11817445486644690944, 11817446517436844544, 11817445486668087296, 11817446517436841984, 11817445486644690944, 11817446517436841984, 11817445486644690944, 11817445488739790818, 11817726961621401602, 11817445490939658239, 11817446521731743746, 11817445490022484036, 11817446517571452929, 11817445486778910212, 11817446517436907522, 11817445490022484036, 11817446517604614500, 11817445486644690944, 11817446517436844544, 11817445486668087296, 11817446517436841984, 11817445486644690944, 11817446517436841984, 11817445486644690944, 11817445488739790818, 11817726961621401602] format="%.0x"
  out "Debug FIFO 2":u32[](array[numeric])=[1, 3, 43680, 1, 3, 43680] format="%.0x"
  out "Debug FIFO 1":u32[](array[numeric]) format="%.0x"
  out "Response":u8[](array[numeric]) format="%.0x"
  out "In Payload":u8[](array[numeric]) format="%.0x"
  in  "Clear Debug FIFOS?":bool
  in  "AXI_STR_RXD_3_tkeep":u8=15
  out "GPIO #1 out":u32 format="%.0x"
  in  "GPIO #2 in":u32=6 format="%.0x"
  in  "GPIO #1 in":u32=6 format="%.0x"
  out "GPIO #2 out":u32=4294967295 format="%.0x"
  out "sPort0_Power_Good":bool=TRUE
  out "signal_detect_Port0":bool=TRUE
  out "aBlockLockPort0":bool=TRUE
  out "UART Receive":string
  out "FPGA Ready":bool
  in  "Read/Write GPIO":bool
  out "error out":errorcluster
  out "Status":string="\r\n"
  in  "error in":errorcluster
  in  "Exit":bool
  in  "Transmit Packet":bool
  in  "Read Packet":bool
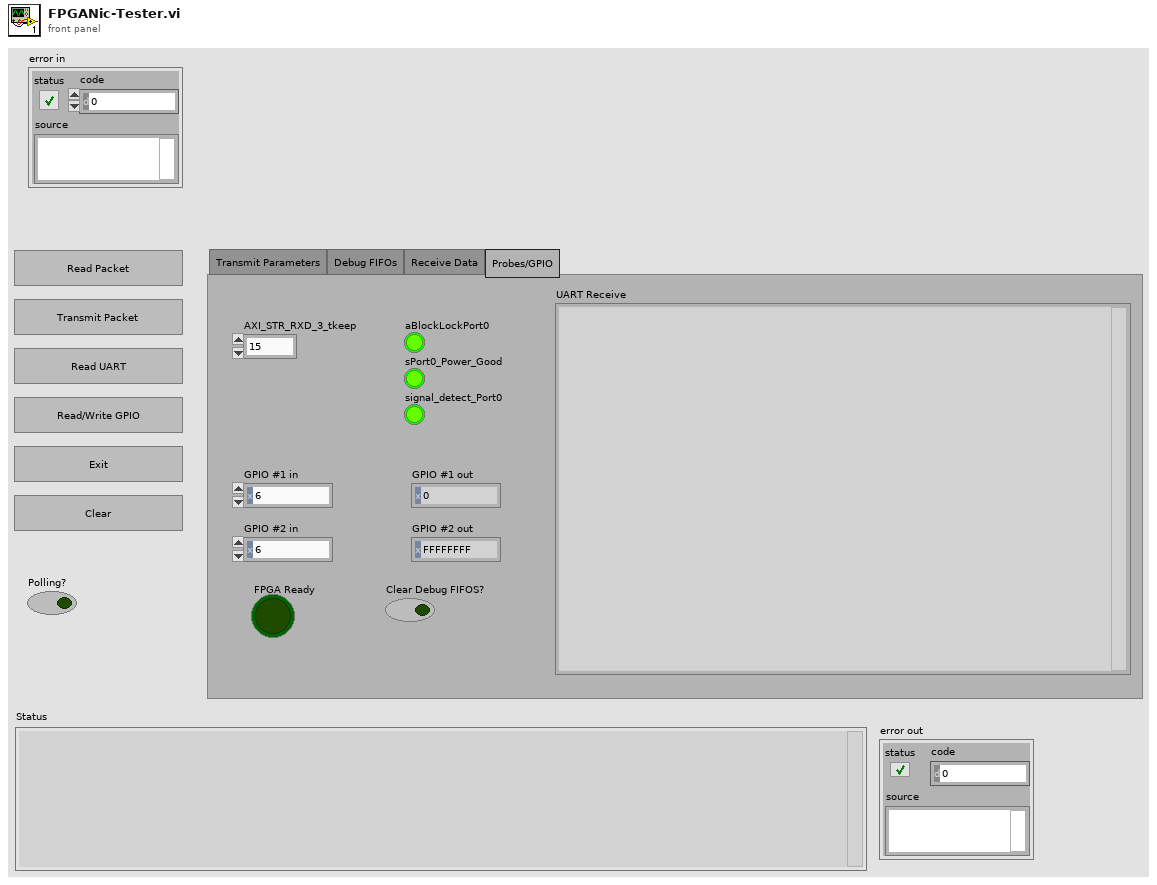
[diagram p1: front panel]
types:
  T1 = enum32{"Transmit Parameters", "Debug FIFOs", "Receive Data", "Probes/GPIO"}
  T2 = cluster{"Destination MAC":u8[], "Source MAC":u8[], "EtherType":u16}
  T3 = cluster{"Destination IP":u8[], "Source IP":u8[], "Protocol":u8}
  T4 = cluster{"Source Port":u16, "Destination Port":u16, "Payload":string}
  T5 = typedef "Source.Machine.Settings.ctl" = cluster{"MAC Address":u8[], "IP Address":u8[]}
  T6 = typedef "FPGANic.Events.ctl" = enum16{"Open FPGA", "Close FPGA", "Reset UI", "Read Packet", "Transmit Packet", "Read UART", "Read Probes", "Read/Write GPIO"}
  T7 = cluster{"Read Probe":u64[], "Write Probe 1":u64[], "Write Probe 2":u64[], "Debug FIFO 1":u32[], "Debug FIFO 2":u32[]}
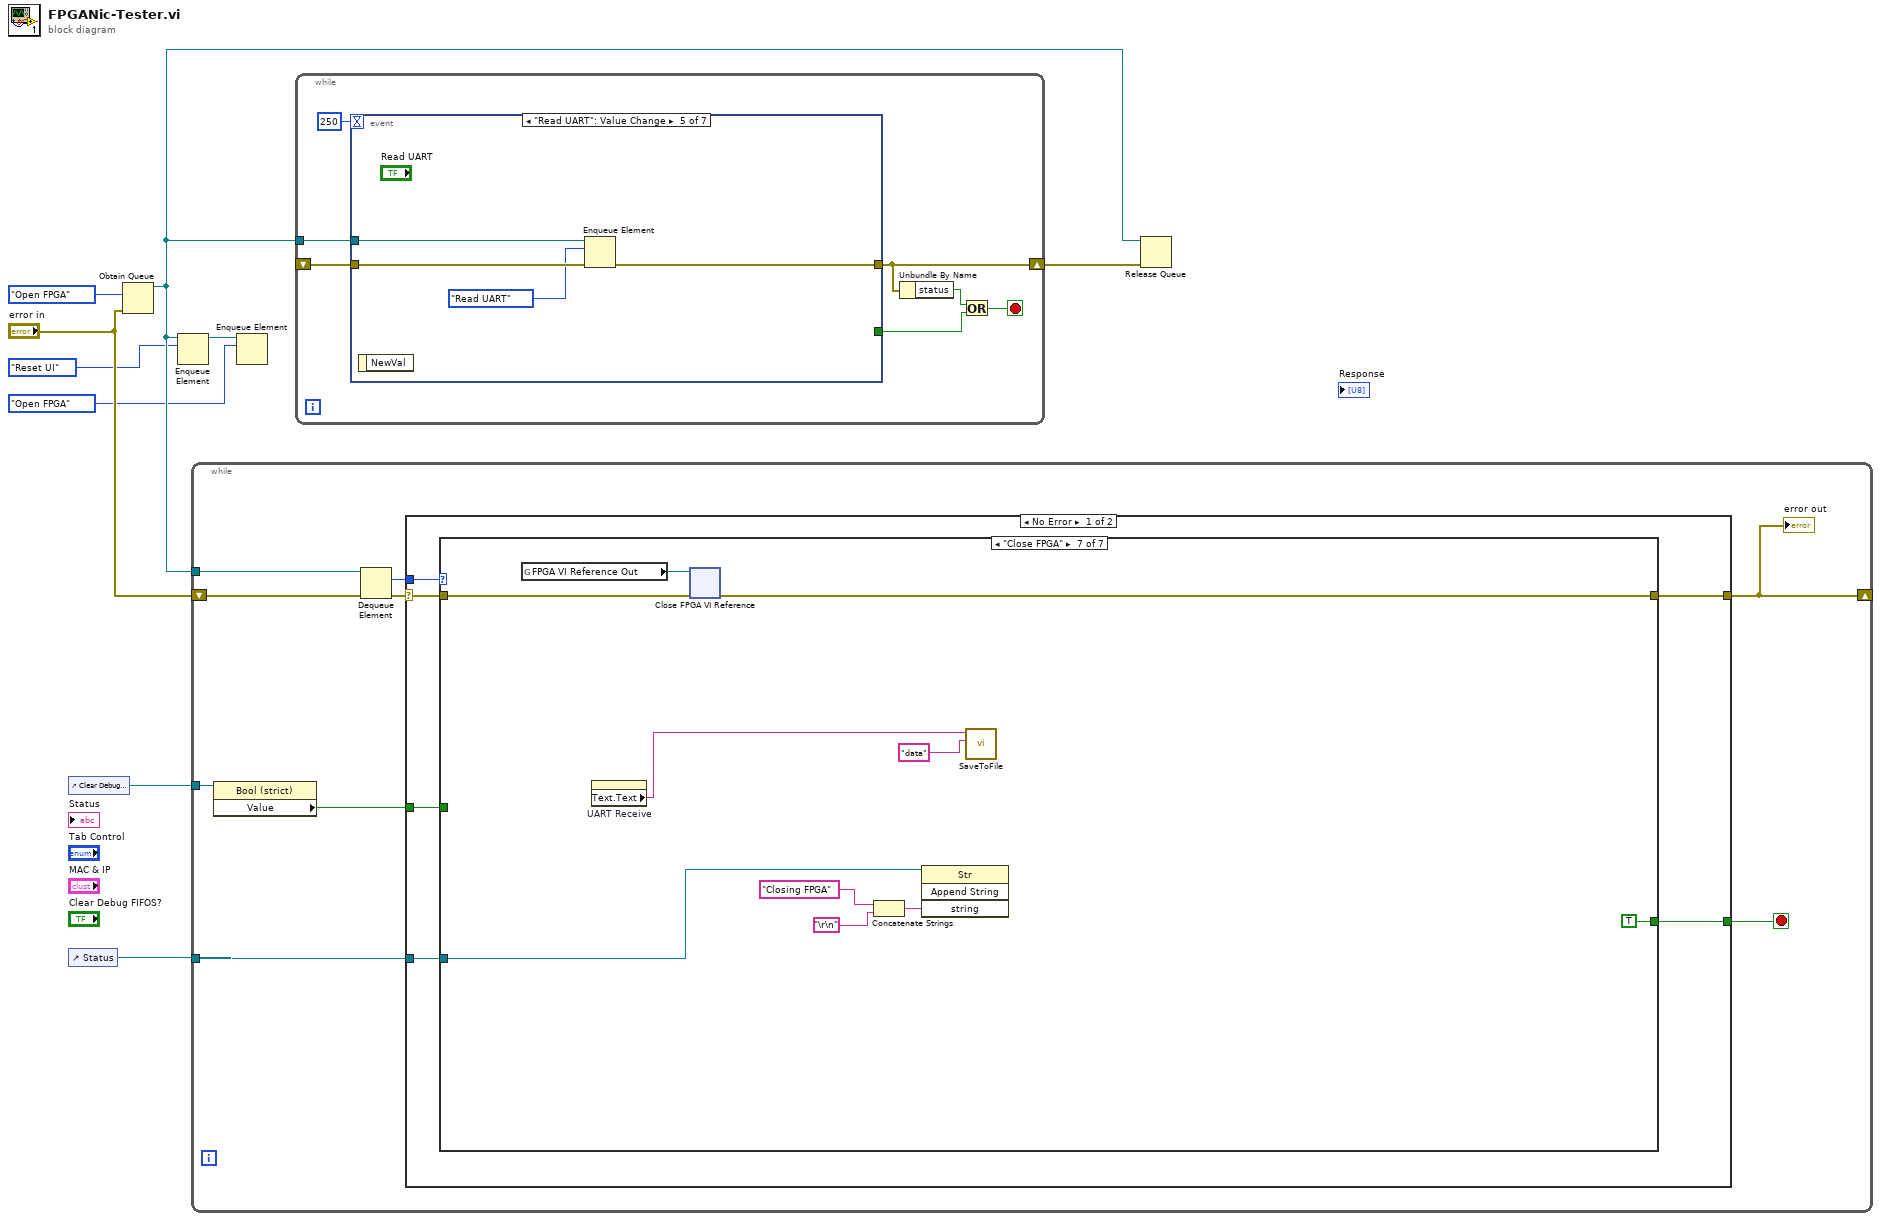
[diagram p0: block diagram]
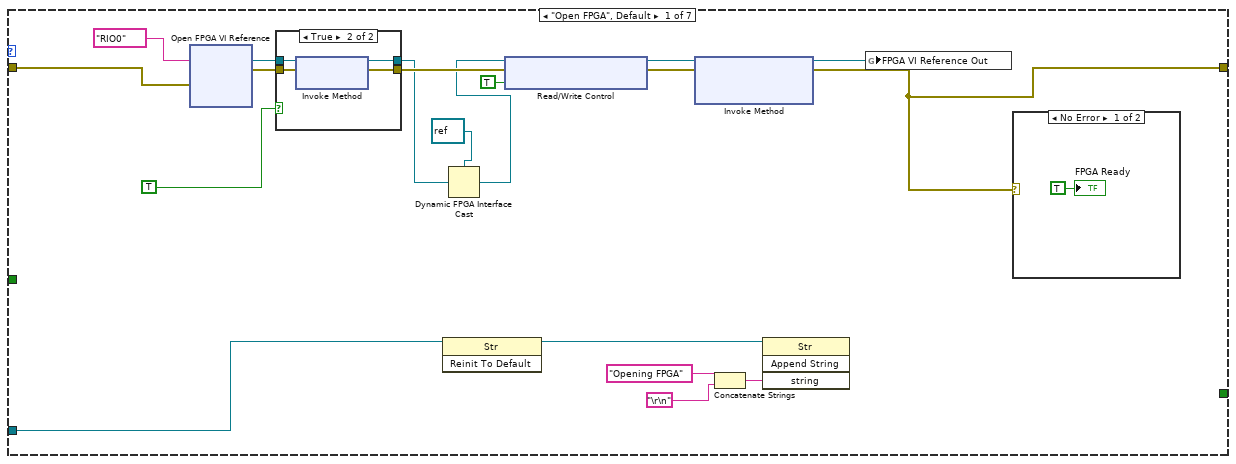
[diagram p2: hidden frame]
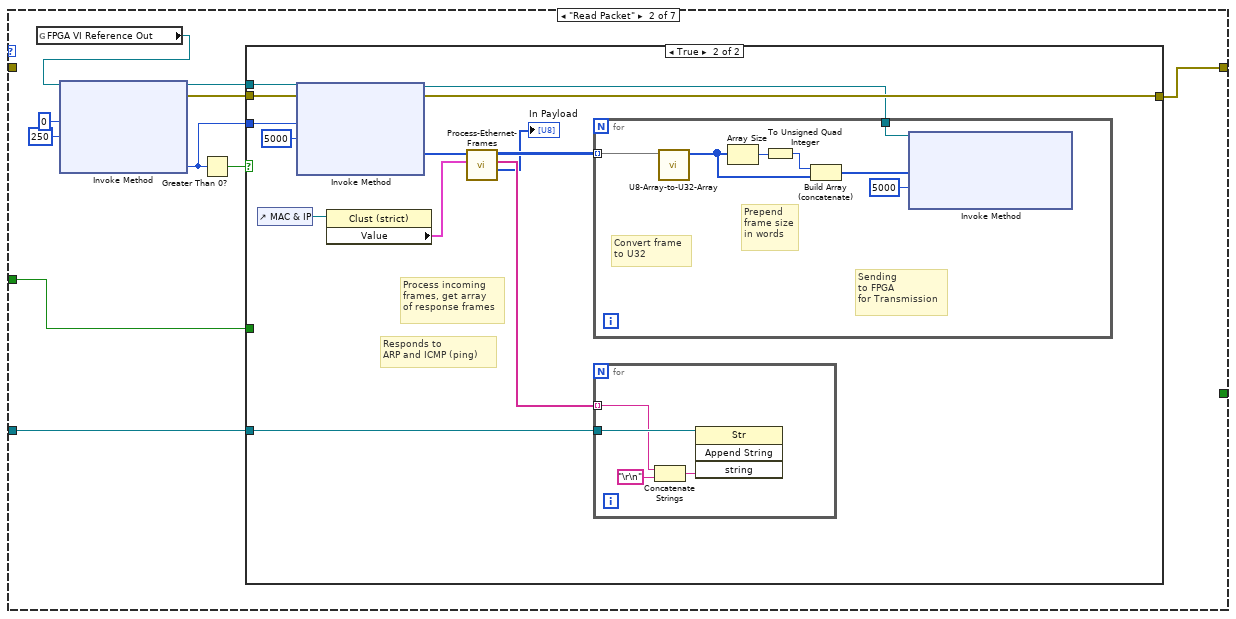
[diagram p5: hidden frame]
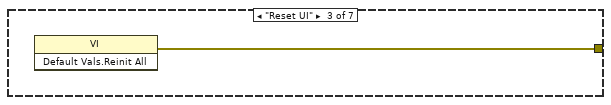
[diagram p7: hidden frame]
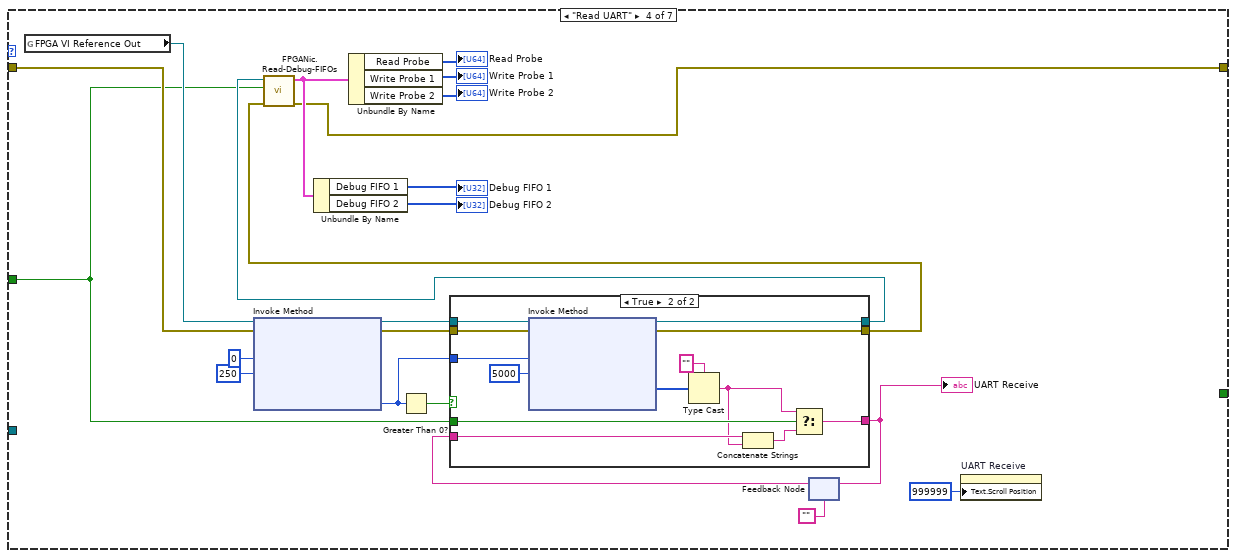
[diagram p8: hidden frame]
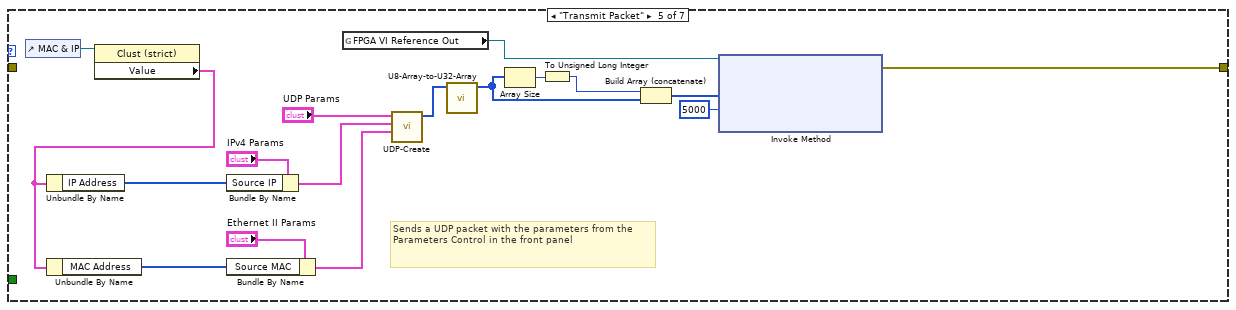
[diagram p10: hidden frame]
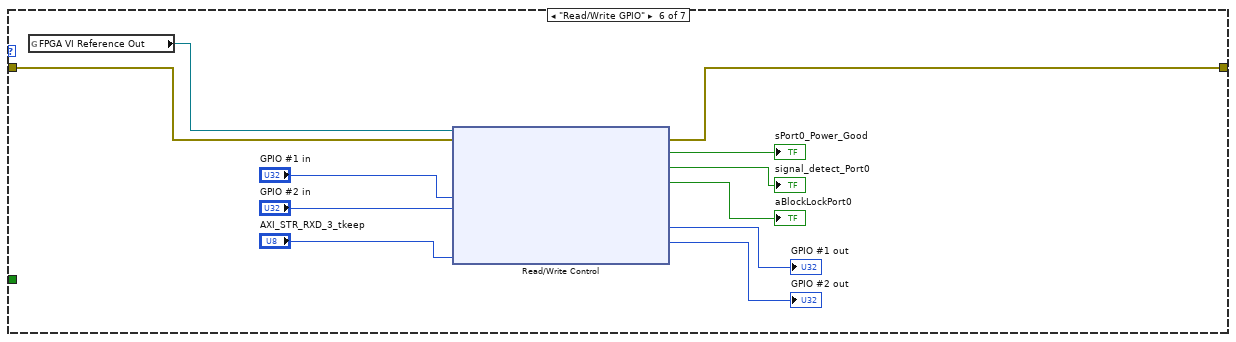
[diagram p11: hidden frame]
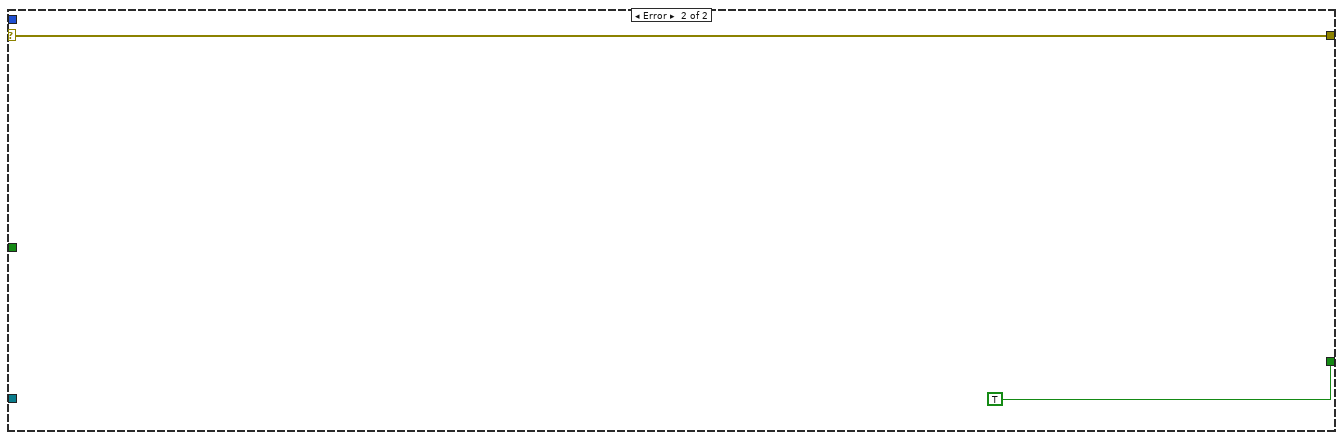
[diagram p12: hidden frame]
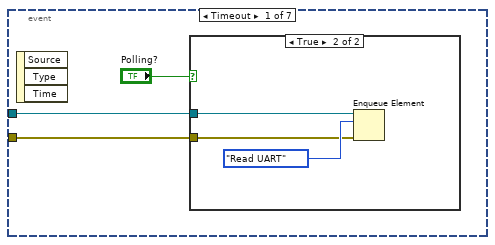
[diagram p13: hidden frame]
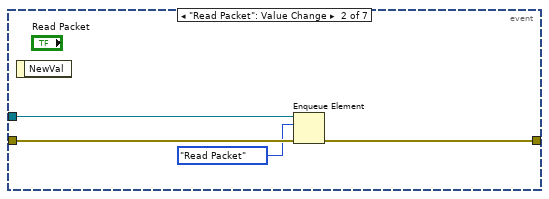
[diagram p15: hidden frame]
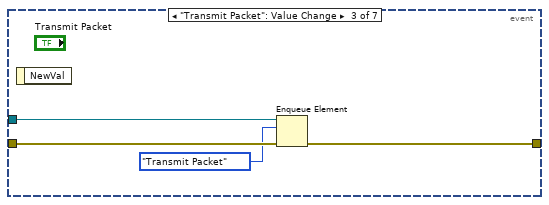
[diagram p16: hidden frame]
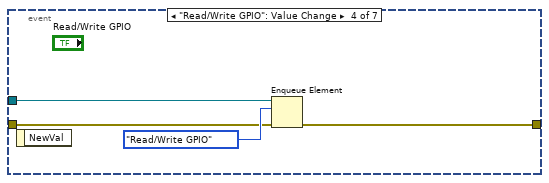
[diagram p17: hidden frame]
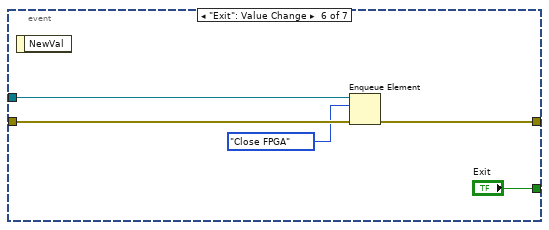
[diagram p18: hidden frame]
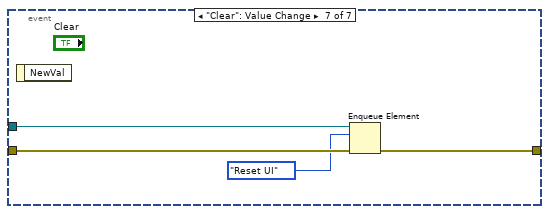
[diagram p19: hidden frame]
diagram:
  n1 = control-ref of="Clear Debug FIFOS?"() -> (w4:refnum<vi>)
  n2 = control-ref of="Status"() -> (w5:refnum<vi>)
  n3 = Obtain Queue(element data type=FPGANic.Events."Open FPGA" ("Enum"), error in (no error)="error in") -> (queue out=w7:refnum<queue>)  [unwired: 3 in, 2 out]
  n4 = Enqueue Element(queue=w7, element=FPGANic.Events."Reset UI" ("Enum")) -> (queue out=w3:refnum<queue>)  [unwired: 2 in, 2 out]
  n5 = while {
    tunnel: w7 -> [w18]
    shift-right: [w13] -> _
    shift-left: "error in" -> [w14]
    tunnel: w5 -> [w12]
    tunnel: w4 -> [w11]
    stop <- w15 stop-if-true
    n6 = property class="Bool (strict)"(reference=w11) -> ("Value"=w10:bool)  [unwired: 1 in, 2 out]
    n7 = Dequeue Element(queue=w18, error in (no error)=w14) -> (element=w16:T6, error out=w17:errorcluster)  [unwired: 1 in, 2 out]
    n8 = case shown="No Error" w17 {
      selector: w17 -> [w19 w163]
      tunnel: w16 -> [w24 _]
      tunnel: [w23 TRUE] -> w15
      tunnel: [w22 w163] -> w13
      tunnel: w12 -> [w21 _]
      tunnel: w10 -> [w20 _]
      frame No Error {
        n9 = case shown="\"Close FPGA\"" w24 {
          tunnel: [_ _ _ _ _ _ TRUE] -> w23
          tunnel: [w30 w55 w86 w90 w139 w144 w161] -> w22
          tunnel: w21 -> [w40 w51 _ _ _ _ w157]
          tunnel: w20 -> [_ w53 _ w96 _ _ _]
          tunnel: w19 -> [w37 _ _ w98 _ w142 w155]
          frame "Open FPGA", Default {
            n10 = xnode "Open FPGA VI Reference"("error in"=w37, "resource name"=tag "RIO0") -> ("FPGA VI Reference Out"=w36:refnum<k20>, "error out"=w35:errorcluster)
            n11 = case shown="True" TRUE ("Download Bitfile?") {
              tunnel: w36 -> [w44 w49]
              tunnel: [w44 w48] -> w25
              tunnel: w35 -> [w45 w47]
              tunnel: [w45 w46] -> w33
              frame False {
              }
              frame True {
                n12 = xnode "Invoke Method"("FPGA VI Reference In"=w49, "error in"=w47) -> ("FPGA VI Reference Out"=w48:refnum<k20>, "error out"=w46:errorcluster)
              }
            }
            n13 = invoke class="Str" method="Reinit To Default"(reference=w40) -> (reference out=w39:refnum<vi>)  [unwired: 2 in, 2 out]
            n14 = Dynamic FPGA Interface Cast(Session In=refnum<k20> refnum ("FPGA VI Reference Out"), Type=w25) -> (Session Out=w26:refnum<k20>)
            n15 = xnode "Read/Write Control"("FPGA VI Reference In"=w26, "error in"=w33, "d_microblaze_i\\reset_rtl"=TRUE ("d_microblaze_i\\reset_rtl")) -> ("FPGA VI Reference Out"=w34:refnum<k20>, "error out"=w31:errorcluster)
            n16 = xnode "Invoke Method"("FPGA VI Reference In"=w34, "error in"=w31) -> ("FPGA VI Reference Out"=w32:refnum<k20>, "error out"=w30:errorcluster)  [unwired: 1 in]
            n17 = Concatenate Strings("Opening FPGA" ("string"), "\r\n") -> (w43:string)
            n18 = invoke class="Str" method="Append String"(reference=w39, "string"=w43) -> ()  [unwired: 2 in, 4 out]
            n19 = global write "FPGANic.Globals.vi" "FPGA VI Reference Out"(w32) -> ()
            n20 = case shown="No Error" w30 {
              frame No Error {
                "FPGA Ready" <- TRUE
              }
              frame Error {
              }
            }
          }
          frame "Read Packet" {
            n21 = global read "FPGANic.Globals.vi" "FPGA VI Reference Out"() -> (w52:refnum<k20>)
            n22 = xnode "Invoke Method"("FPGA VI Reference In"=w52, "Number of Elements"=u32 0, "Timeout (ms)"=250) -> ("FPGA VI Reference Out"=w57:refnum<k20>, "error out"=w56:errorcluster, "Elements Remaining"=w54:u32)  [unwired: 1 in, 1 out]
            n23 = Greater Than 0?(x=w54) -> (x > 0?=w58:bool)
            n24 = case shown="True" w58 {
              tunnel: w57 -> [_ w73]
              tunnel: w56 -> [w61 w72]
              tunnel: [w61 w70] -> w55
              tunnel: w54 -> [_ w71]
              tunnel: w53 -> [_ _]
              tunnel: w51 -> [_ w64]
              frame False {
              }
              frame True {
                # "Responds to\nARP and ICMP (ping)"
                # "Process incoming\nframes, get array\nof response frames"
                n25 = control-ref of="MAC & IP"() -> (w67:refnum<vi>)
                n26 = xnode "Invoke Method"("FPGA VI Reference In"=w73, "error in"=w72, "Number of Elements"=w71, "Timeout (ms)"=5000) -> ("FPGA VI Reference Out"=w65:refnum<k20>, "error out"=w70:errorcluster, "Data"=w69:u64[])  [unwired: 1 out]
                n27 = property class="Clust (strict)"(reference=w67) -> ("Value"=w66:T5)  [unwired: 1 in, 2 out]
                n28 = call "Process-Ethernet-Frames.vi"("Source Machine\nSettings"=w66, "Raw Data\nStream"=w69) -> ("UDP Payload"=→"In Payload":u8[], "Messages"=w63:string[], "Frames to send"=w68:u8[][])  [unwired: 7 in]
                n29 = for {
                  tunnel: w68 -> [w85] mode=indexing
                  tunnel: w65 -> [w79]
                  # "Prepend\nframe size\nin words"
                  # "Sending\nto FPGA\nfor Transmission"
                  # "Convert frame\nto U32"
                  n30 = call "U8-Array-to-U32-Array.vi"("Frame U8[] in"=w85) -> ("Frame U32[] out"=w80:u32[])  [unwired: 10 in]
                  n31 = Array Size(array=w80) -> (size(s)=w84:i32)
                  n32 = To Unsigned Quad Integer(1:w84) -> (0:w83:u64)
                  n33 = Build Array (concatenate)(w83, w80) -> (w82:u64[])
                  n34 = xnode "Invoke Method"("FPGA VI Reference In"=w79, "Data"=w82, "Timeout (ms)"=5000) -> ()  [unwired: 1 in, 3 out]
                }
                n35 = for {
                  tunnel: w64 -> [w76]
                  tunnel: w63 -> [w75] mode=indexing
                  n36 = Concatenate Strings(w75, "\r\n") -> (w78:string)
                  n37 = invoke class="Str" method="Append String"(reference=w76, "string"=w78) -> ()  [unwired: 2 in, 4 out]
                }
              }
            }
          }
          frame "Reset UI" {
            n38 = invoke class="VI" method="Default Vals.Reinit All"() -> (error out=w86:errorcluster)  [unwired: 3 in, 2 out]
          }
          frame "Read UART" {
            n39 = global read "FPGANic.Globals.vi" "FPGA VI Reference Out"() -> (w99:refnum<k20>)
            n40 = xnode "Invoke Method"("FPGA VI Reference In"=w99, "error in"=w98, "Number of Elements"=u32 0, "Timeout (ms)"=250) -> ("FPGA VI Reference Out"=w106:refnum<k20>, "error out"=w105:errorcluster, "Elements Remaining"=w102:u32)  [unwired: 1 out]
            n41 = Greater Than 0?(x=w102) -> (x > 0?=w104:bool)
            n42 = feedback #1("") -> (w103:string)
            n43 = case shown="True" w104 {
              tunnel: w103 -> [w111 w124]
              tunnel: w102 -> [_ w123]
              tunnel: w105 -> [w110 w121]
              tunnel: w106 -> [w109 w120]
              tunnel: [w111 w115] -> w100
              tunnel: [w110 w119] -> w95
              tunnel: w96 -> [_ w117]
              tunnel: [w109 w112] -> w97
              frame False {
              }
              frame True {
                n44 = xnode "Invoke Method"("FPGA VI Reference In"=w120, "error in"=w121, "Number of Elements"=w123, "Timeout (ms)"=5000) -> ("FPGA VI Reference Out"=w112:refnum<k20>, "error out"=w119:errorcluster, "Data"=w114:u8[])  [unwired: 1 out]
                n45 = Type Cast(type="", x=w114) -> (*(type *) &x=w113:string)
                n46 = Concatenate Strings(w124, w113) -> (w118:string)
                n47 = Select(t=w113, s=w117, f=w118) -> (s? t:f=w115:string)
              }
            }
            "UART Receive" <- w100
            n48 = call "FPGANic.Read-Debug-FIFOs.vi"("error in"=w95, "Clear Debug FIFOs"=w96, "FPGA VI Reference In"=w97) -> ("error out"=w90:errorcluster, "Debug Data"=w93:T7)  [unwired: 7 in]
            n49 = Unbundle By Name(w93) -> ("Debug FIFO 1"=→"Debug FIFO 1":u32[], "Debug FIFO 2"=→"Debug FIFO 2":u32[])
            n50 = Unbundle By Name(w93) -> ("Read Probe"=→"Read Probe":u64[], "Write Probe 1"=→"Write Probe 1":u64[], "Write Probe 2"=→"Write Probe 2":u64[])
            n51 = feedback-in #1(w100) -> ()
            n52 = property on="UART Receive" class="Str"("Text.Scroll Position"=u32 999999) -> ()  [unwired: 2 in, 2 out]
          }
          frame "Transmit Packet" {
            # "Sends a UDP packet with the parameters from the\nParameters Control in the front panel"
            n53 = control-ref of="MAC & IP"() -> (w128:refnum<vi>)
            n54 = property class="Clust (strict)"(reference=w128) -> ("Value"=w126:T5)  [unwired: 1 in, 2 out]
            n55 = Unbundle By Name(w126) -> ("IP Address"=w127:u8[])
            n56 = Unbundle By Name(w126) -> ("MAC Address"=w125:u8[])
            n57 = Bundle By Name(cluster="IPv4 Params", "Source IP"=w127) -> (w129:T3)
            n58 = Bundle By Name(cluster="Ethernet II Params", "Source MAC"=w125) -> (w130:T2)
            n59 = global read "FPGANic.Globals.vi" "FPGA VI Reference Out"() -> (w138:refnum<k20>)
            n60 = call "UDP-Create.vi"("Ethernet II Params"=w130, "IPv4 Params"=w129, "UDP Params"="UDP Params") -> ("Ethernet Frame"=w137:u8[])  [unwired: 6 in, 2 out]
            n61 = call "U8-Array-to-U32-Array.vi"("Frame U8[] in"=w137) -> ("Frame U32[] out"=w134:u32[])  [unwired: 10 in]
            n62 = Array Size(array=w134) -> (size(s)=w136:i32)
            n63 = To Unsigned Long Integer(number=w136) -> (unsigned 32bit integer=w135:u32)
            n64 = Build Array (concatenate)(w135, w134) -> (w133:u32[])
            n65 = xnode "Invoke Method"("FPGA VI Reference In"=w138, "Data"=w133, "Timeout (ms)"=5000) -> ("error out"=w139:errorcluster)  [unwired: 1 in, 2 out]
          }
          frame "Read/Write GPIO" {
            n66 = global read "FPGANic.Globals.vi" "FPGA VI Reference Out"() -> (w143:refnum<k20>)
            n67 = xnode "Read/Write Control"("FPGA VI Reference In"=w143, "error in"=w142, "GPIO #1 in"="GPIO #1 in", "GPIO #2 in"="GPIO #2 in", "d_microblaze_i\\AXI_STR_RXD_3_tkeep"="AXI_STR_RXD_3_tkeep") -> ("error out"=w144:errorcluster, "sPort0_Power_Good"=→"sPort0_Power_Good":bool, "signal_detect_Port0"=→"signal_detect_Port0":bool, "aBlockLockPort0"=→"aBlockLockPort0":bool, "GPIO #1 out"=→"GPIO #1 out":u32, "GPIO #2 out"=→"GPIO #2 out":u32)  [unwired: 1 out]
          }
          frame "Close FPGA" {
            n68 = global read "FPGANic.Globals.vi" "FPGA VI Reference Out"() -> (w156:refnum<k20>)
            n69 = property on="UART Receive" class="Str"() -> ("Text.Text"=w154:string)  [unwired: 2 in, 2 out]
            n70 = xnode "Close FPGA VI Reference"("FPGA VI Reference In"=w156, "error in"=w155) -> ("error out"=w161:errorcluster)
            n71 = Concatenate Strings("Closing FPGA" ("string"), "\r\n") -> (w160:string)
            n72 = invoke class="Str" method="Append String"(reference=w157, "string"=w160) -> ()  [unwired: 2 in, 4 out]
            n73 = call "SaveToFile.vi"("FileNamePrefix"="data" ("Text.Text"), "TextToWrite"=w154) -> ()  [unwired: 10 in]
          }
        }
      }
      frame Error {
      }
    }
    "error out" <- w13
  }
  n74 = Enqueue Element(queue=w3, element=FPGANic.Events."Open FPGA" ("Enum")) -> ()  [unwired: 2 in, 3 out]
  n75 = while {
    tunnel: w7 -> [w171]
    shift-right: [w166] -> w8
    shift-left: _ -> [w167]
    stop <- w169 stop-if-true
    n76 = event shown="[4] \"Read UART\": Value Change" {
      selector: _ -> [_ _ _ _ _ _ _]
      dyn-events: _ -> [_ _ _ _ _ _ _]
      timeout: 250 -> [_ _ _ _ _ _ _]
      tunnel: w171 -> [w174 w181 w185 w188 w193 w198 w202]
      tunnel: [_ w180 w183 w186 w190 w197 w201] -> w166
      tunnel: [_ _ _ _ _ "Exit" _] -> w168
      tunnel: w167 -> [w173 w179 w184 w187 w192 w195 w200]
      event Timeout {
        n77 = event-data() -> ()  [unwired: 1 in, 3 out]
        n78 = case shown="True" "Polling?" {
          tunnel: w174 -> [_ w176]
          tunnel: w173 -> [_ w175]
          frame False {
          }
          frame True {
            n79 = Enqueue Element(queue=w176, element=FPGANic.Events."Read UART" ("Enum"), error in (no error)=w175) -> ()  [unwired: 1 in, 3 out]
          }
        }
      }
      event "Read Packet": Value Change {
        n80 = event-data() -> ()  [unwired: 1 in, 1 out]
        n81 = Enqueue Element(queue=w181, element=FPGANic.Events."Read Packet" ("Enum"), error in (no error)=w179) -> (error out=w180:errorcluster)  [unwired: 1 in, 2 out]
      }
      event "Transmit Packet": Value Change {
        n82 = event-data() -> ()  [unwired: 1 in, 1 out]
        n83 = Enqueue Element(queue=w185, element=FPGANic.Events."Transmit Packet" ("Enum"), error in (no error)=w184) -> (error out=w183:errorcluster)  [unwired: 1 in, 2 out]
      }
      event "Read/Write GPIO": Value Change {
        n84 = event-data() -> ()  [unwired: 1 in, 1 out]
        n85 = Enqueue Element(queue=w188, element=FPGANic.Events."Read/Write GPIO" ("Enum"), error in (no error)=w187) -> (error out=w186:errorcluster)  [unwired: 1 in, 2 out]
      }
      event "Read UART": Value Change {
        n86 = event-data() -> ()  [unwired: 1 in, 1 out]
        n87 = Enqueue Element(queue=w193, element=FPGANic.Events."Read UART" ("Enum"), error in (no error)=w192) -> (error out=w190:errorcluster)  [unwired: 1 in, 2 out]
      }
      event "Exit": Value Change {
        n88 = event-data() -> ()  [unwired: 1 in, 1 out]
        n89 = Enqueue Element(queue=w198, element=FPGANic.Events."Close FPGA" ("Enum"), error in (no error)=w195) -> (error out=w197:errorcluster)  [unwired: 1 in, 2 out]
      }
      event "Clear": Value Change {
        n90 = event-data() -> ()  [unwired: 1 in, 1 out]
        n91 = Enqueue Element(queue=w202, element=FPGANic.Events."Reset UI" ("Enum"), error in (no error)=w200) -> (error out=w201:errorcluster)  [unwired: 1 in, 2 out]
      }
    }
    n92 = Unbundle By Name(w166) -> ("status"=w170:bool)
    n93 = Or(x=w170, y=w168) -> (x .or. y?=w169:bool)
  }
  n94 = Release Queue(queue=w7, error in (no error)=w8) -> ()  [unwired: 1 in, 3 out]
